vi "RIO_or_DAQ Update control bounds and format.vi"(10 "RIO? in":bool, 11 "Control References in":refnum<vi>[](array[refnum])) -> ()   [LabVIEW 2013]
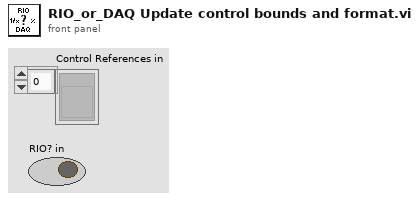
[diagram p1: front panel]
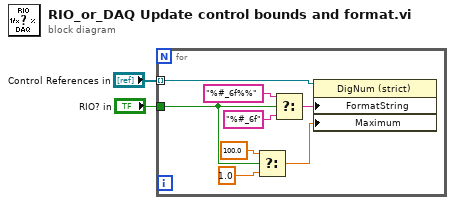
[diagram p0: block diagram]
diagram:
  n1 = for {
    tunnel: "RIO? in" -> [w8]
    tunnel: "Control References in" -> [w3] mode=indexing
    n2 = Select(t=100.0, s=w8, f=1.0) -> (s? t:f=w10:dbl)
    n3 = Select(t="%#_6f%%", s=w8, f="%#_6f") -> (s? t:f=w9:string)
    n4 = property on="Property Node" class="DigNum (strict)"(reference=w3, "FormatString"=w9, "Maximum"=w10) -> ()  [unwired: 1 in, 2 out]
  }
